vi "sub_initializeTopLevelQueue.vi"(9 "list of guesses":T1[](array[typedef]), 11 "Q1":refnum<queue>) -> ()   [LabVIEW 2018]
uses:
  guess.ctl
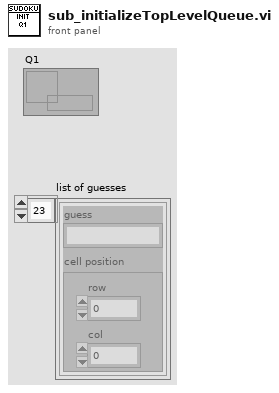
[diagram p1: front panel]
types:
  T1 = typedef "guess.ctl" = cluster{"cell position":cluster{"row":i32, "col":i32}, "guess":string}
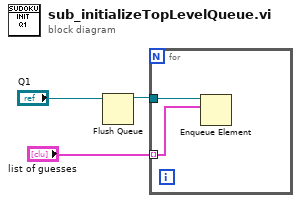
[diagram p0: block diagram]
diagram:
  n1 = Flush Queue(queue="Q1") -> (queue out=w1:refnum<queue>)  [unwired: 1 in, 2 out]
  n2 = for {
    tunnel: "list of guesses" -> [w5] mode=indexing
    tunnel: w1 -> [w4]
    n3 = Enqueue Element(queue=w4, element=w5) -> ()  [unwired: 2 in, 3 out]
  }
